vi "Execute.vi"(8 "Error In":errorcluster, 9 "Workspace":T1, 10 "Control In":T2={"I-O.lvclass"=refnum, "Motion.lvclass"=refnum, "Dispenser.lvclass"=refnum}, 11 "Dispense in":refnum<class "Dispense.lvclass">) -> (0 "Error Out":errorcluster, 2 "Control Out":T2, 3 "Dispense in 2":refnum<class "Dispense.lvclass">)   [LabVIEW 2016, in "Dispense.lvclass"]
uses:
  Dispense.lvclass
  Controller/Controllers.ctl
  Controller/I-O/I-O.lvclass
  Controller/Motion/A3200/A3200.lvclass
  Controller/Dispenser/Dispenser.lvclass
  Controller/Motion/Motion.lvclass
  Workspace/Workspace.ctl
  Dispense.lvclass/Dispense.ctl
  Controller/Motion/Motion.lvclass/Motion.ctl
  Controller/Motion/Read XYAcceleration.vi
  Controller/Controller.lvclass
  Workspace/Fixture.lvclass
panel:
  out "error out":errorcluster
  out "XYZTheta 2":dbl[](array[numeric])
  out "XYZTheta":dbl[](array[numeric])
  out "Pattern Coordinates":dbl[][](array[numeric])
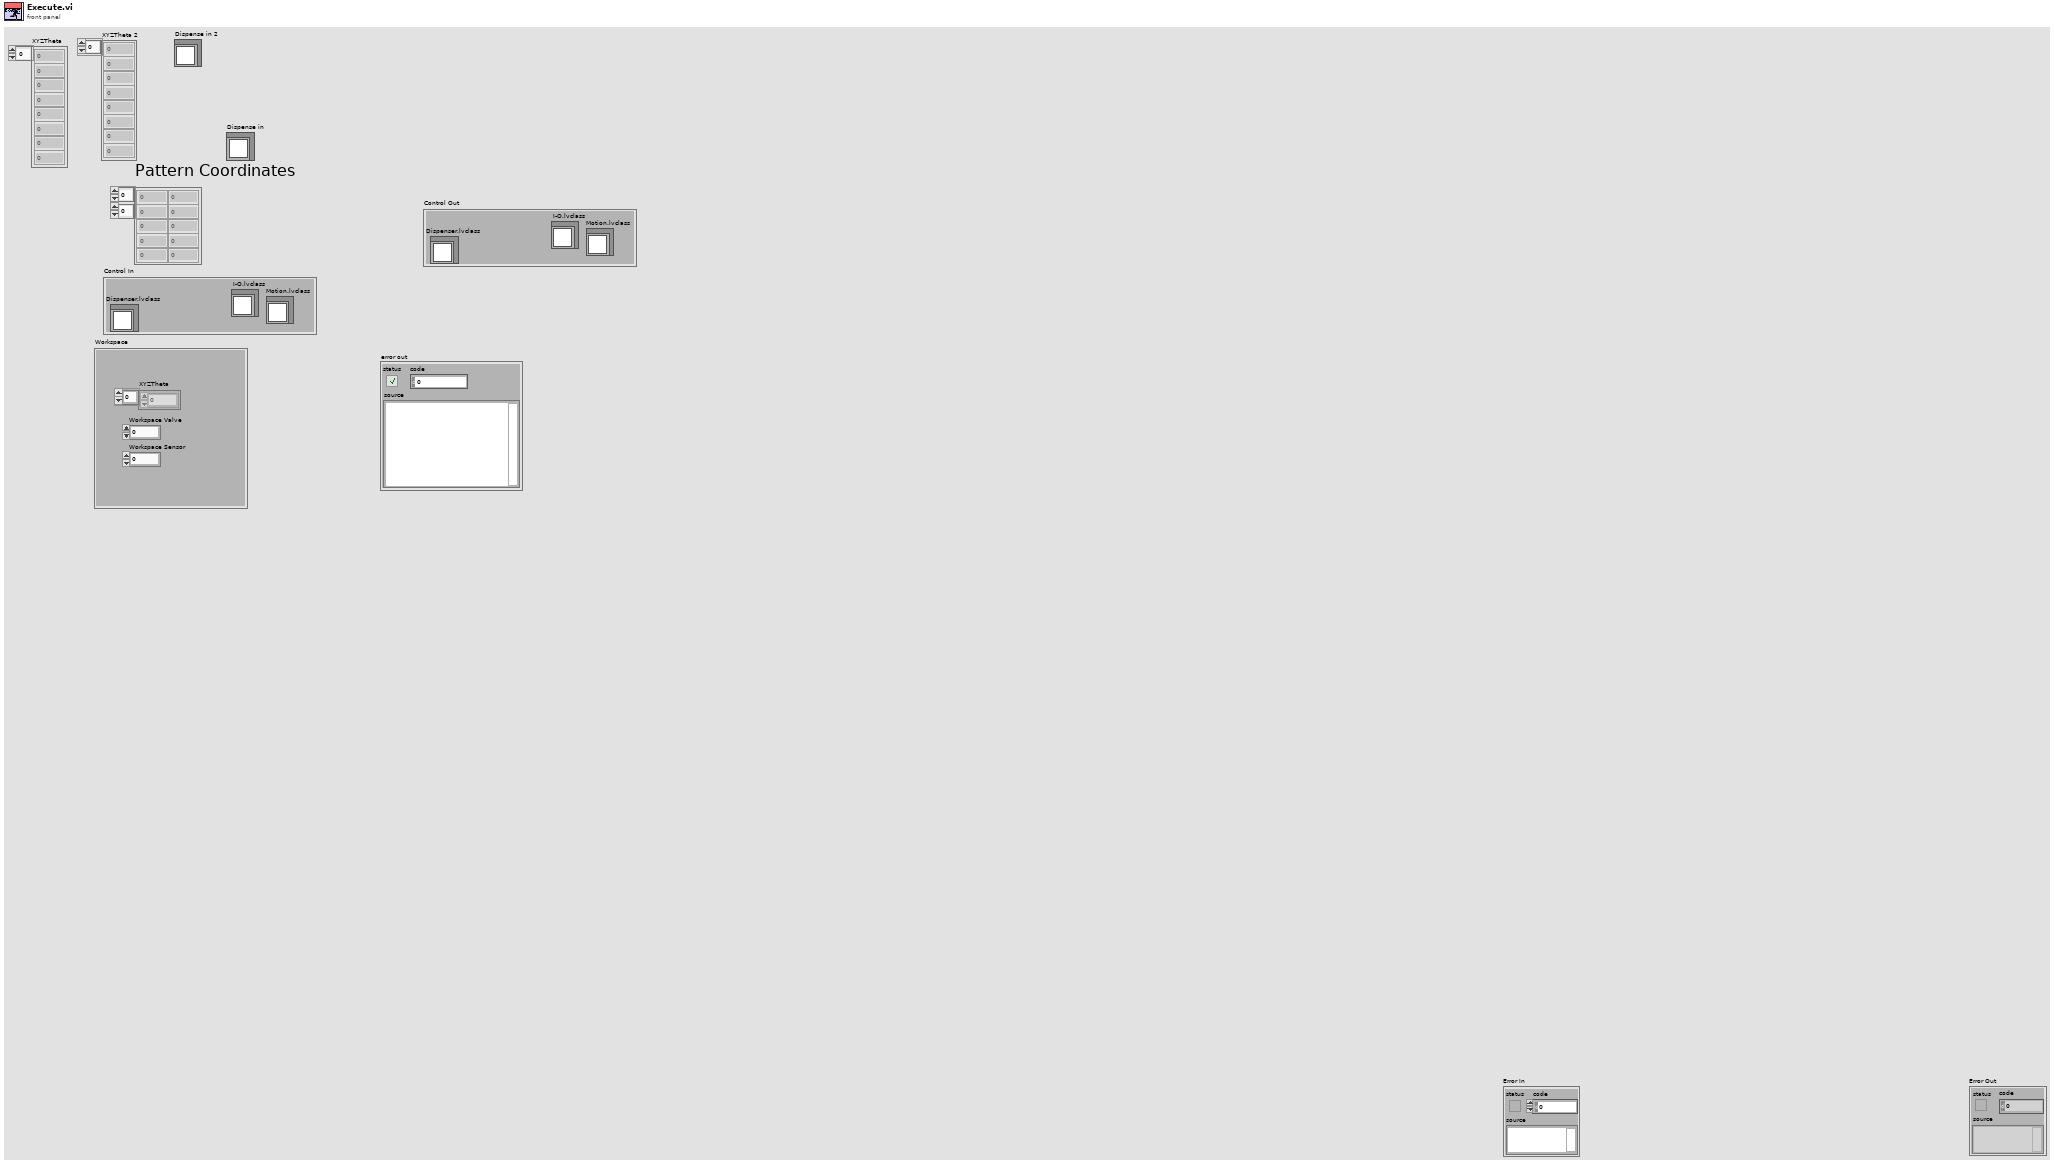
[diagram p1: front panel]
types:
  T1 = typedef "Fixture.lvclass/Workspace.ctl" = cluster{"XYZTheta":dbl[], "Workspace Valve":i32, "Workspace Sensor":i32}
  T2 = typedef "Controller.lvclass/Controllers.ctl" = cluster{"I-O.lvclass":refnum<class "I-O.lvclass">, "Motion.lvclass":refnum<class "Motion.lvclass">, "Dispenser.lvclass":refnum<class "Dispenser.lvclass">}
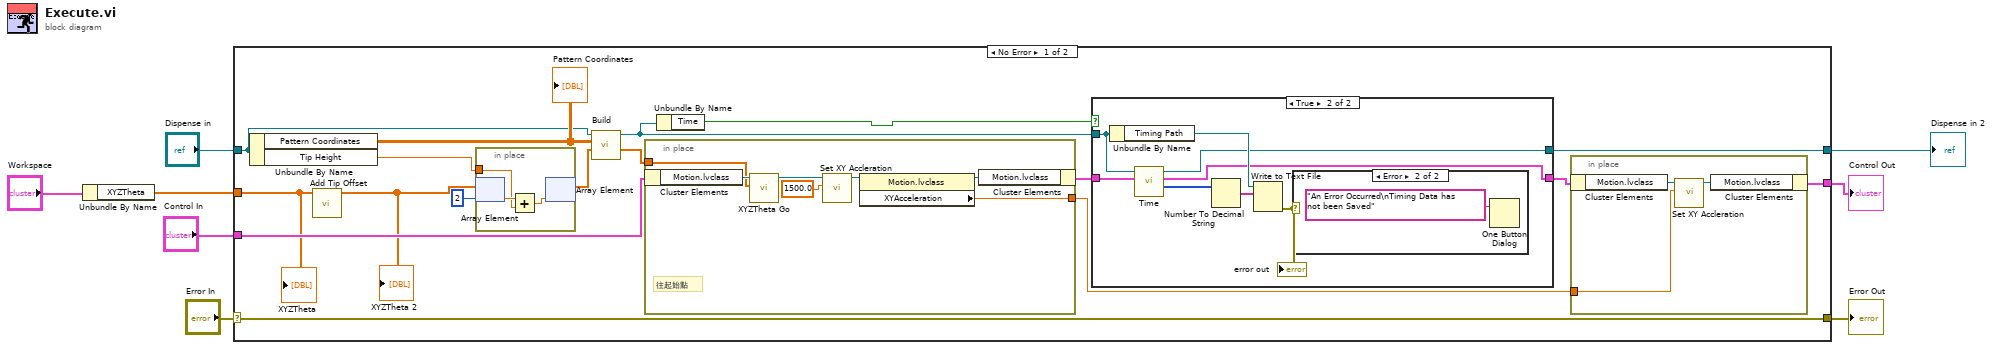
[diagram p0: block diagram]
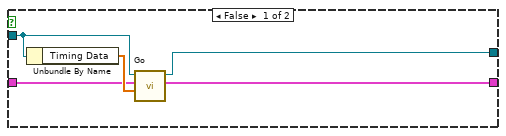
[diagram p2: hidden frame]
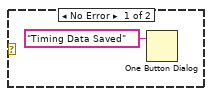
[diagram p3: hidden frame]
diagram:
  n1 = Unbundle By Name("Workspace") -> ("XYZTheta"=w2:dbl[])
  n2 = case shown="No Error" "Error In" {
    selector: "Error In" -> [w25 w55]
    tunnel: "Control In" -> [w17 w56]
    tunnel: [w11 w56] -> w7
    tunnel: "Dispense in" -> [w16 w54]
    tunnel: [w25 w55] -> w4
    tunnel: w2 -> [w15 _]
    tunnel: [w23 w54] -> w1
    frame No Error {
      n3 = Unbundle By Name(w16) -> ("Pattern Coordinates"=w21:dbl[][], "Tip Height"=w18:dbl)
      "Pattern Coordinates" <- w21
      n4 = call "Add Tip Offset.vi"("XYZTheta"=w15) -> ("XYZTheta"=w14:dbl[])  [unwired: 10 in]
      "XYZTheta 2" <- w14
      n5 = in-place {
        in-place-border: w18 -> [w29]
        n6 = in-place-array #1(w14, 2) -> (w31:dbl)
        n7 = Add(x=w31, y=w29) -> (x+y=w30:dbl)
        n8 = in-place-array #1(w30) -> (w19:dbl[])  [unwired: 1 out]
      }
      n9 = call-dynamic "Build.vi"("XYZTheta"=w19, "Pattern Coordinates"=w21, "Dispense in"=w16) -> ("Starting Coordinates"=w22:dbl[], "Dispense out"=w24:refnum<class "Dispense.lvclass">)  [unwired: 7 in]
      n10 = in-place {
        in-place-border: w22 -> [w37]
        in-place-border: [w33] -> w10
        # "往起始點"
        n11 = in-place-cluster #2(w17) -> ("Motion.lvclass"=w38:refnum<class "Motion.lvclass">)
        n12 = call "XYZTheta Go.vi"("XYZTheta In"=w37, "Motion in"=w38) -> ("Motion out"=w36:refnum<class "Motion.lvclass">)  [unwired: 7 in, 2 out]
        n13 = call-dynamic "Set XY Accleration.vi"("mm/s"=1500.0, "Motion in"=w36) -> ("Motion out"=w35:refnum<class "Motion.lvclass">)  [unwired: 8 in, 1 out]
        n14 = property class="Motion.lvclass"(reference=w35) -> (reference out=w34:refnum<class "Motion.lvclass">, "XYAcceleration"=w33:dbl)  [unwired: 1 in, 1 out]
        n15 = in-place-cluster #2("Motion.lvclass"=w34) -> (w13:T2)
      }
      n16 = Unbundle By Name(w24) -> ("Time"=w9:bool)
      n17 = case shown="True" w9 {
        tunnel: w24 -> [w40 w45]
        tunnel: w13 -> [w39 w47]
        tunnel: [w43 w46] -> w12
        tunnel: [w41 w44] -> w23
        frame False {
          n18 = Unbundle By Name(w40) -> ("Timing Data"=w42:dbl[])
          n19 = call-dynamic "Go.vi"("Timing Data"=w42, "Control In"=w39, "Dispense in"=w40) -> ("Control Out"=w43:T2, "Dispense Out"=w41:refnum<class "Dispense.lvclass">)  [unwired: 7 in]
        }
        frame True {
          n20 = Unbundle By Name(w45) -> ("Timing Path"=w49:path)
          n21 = call-dynamic "Time.vi"("Control In"=w47, "Dispense in"=w45) -> ("Timing Data"=w48:i32[], "Control Out"=w46:T2, "Dispense out"=w44:refnum<class "Dispense.lvclass">)  [unwired: 6 in, 1 out]
          n22 = Number To Decimal String(number=w48) -> (decimal integer string=w50:string[])  [unwired: 1 in]
          n23 = Write to Text File(file (use dialog)=w49, text=w50) -> (error out=w51:errorcluster)  [unwired: 2 in, 2 out]
          "error out" <- w51
          n24 = case shown="Error" w51 {
            frame No Error {
              n25 = One Button Dialog(message="Timing Data Saved") -> ()  [unwired: 1 in, 1 out]
            }
            frame Error {
              n26 = One Button Dialog(message="An Error Occurred\nTiming Data has not been Saved") -> ()  [unwired: 1 in, 1 out]
            }
          }
        }
      }
      n27 = in-place {
        in-place-border: w10 -> [w26]
        n28 = in-place-cluster #3(w12) -> ("Motion.lvclass"=w28:refnum<class "Motion.lvclass">)
        n29 = call-dynamic "Set XY Accleration.vi"("mm/s"=w26, "Motion in"=w28) -> ("Motion out"=w27:refnum<class "Motion.lvclass">)  [unwired: 8 in, 1 out]
        n30 = in-place-cluster #3("Motion.lvclass"=w27) -> (w11:T2)
      }
      "XYZTheta" <- w15
    }
    frame Error {
    }
  }
  "Control Out" <- w7
  "Error Out" <- w4
  "Dispense in 2" <- w1
